vi "RNN_Backward_Pass_demo_alt.vi"() -> ()   [LabVIEW 2014]
uses:
  <vilib>/Analysis/Matrix/Datatypes/RealMatrix.ctl
  <vilib>/Analysis/baseanly.llb/A x Vector.vi
  <vilib>/Analysis/Matrix/Numeric/Conversions/Array To Matrix - RA.vi
  <vilib>/Analysis/Matrix/Numeric/Add/Add - RM,RM.vi
  <vilib>/Analysis/Matrix/NI_Matrix.lvlib
  <vilib>/Analysis/NI_AALBase.lvlib
panel:
  in  "step through t?":bool
  in  "t --->  t - 1":bool
  out "t":i32
  out "t (reversed)":i32
  out "input length":i32=1
  out "dy":dbl[](array[numeric])=[-0.7971630000000001, 0.104457, 0.692257] format="%_8f"
  out "dhnext (out)":dbl[](array[numeric])=[-0.01793824867590542, 0.021743253148573408] format="%_8f"
  out "dhnext (in)":dbl[](array[numeric]) format="%_8f"
  out "dhraw":dbl[](array[numeric])=[0.001989539982402268, -0.041566378972628285] format="%_8f"
  out "dh":dbl[](array[numeric])=[0.24857070126380001, -0.8002550289340001] format="%_8f"
  out "hs[t]":dbl[](array[numeric])=[0.99599, -0.973683] format="%_8f"
  out "hs[t-1]":dbl[](array[numeric]) format="%_8f"
  out "dby":T1=[[-0.7971630000000001], [0.104457], [0.692257]] format="%_8f"
  out "dbh":T1=[[0.001989539982402268], [-0.041566378972628285]] format="%_8f"
  out "dWhy":T1=[[-0.7939663763700001, 0.7761840613290001], [0.10403812743, -0.10170800513099999], [0.68948104943, -0.674038872531]] format="%_8f"
  out "dWhh":T1 format="%_8f"
  out "dWxh":T1=[[0.0, 0.001989539982402268, 0.0], [0.0, -0.041566378972628285, 0.0]] format="%_8f"
  in  "by":T1=[[-0.528417], [-0.44032], [-0.8844819]] format="%_8f"
  in  "bh":T1=[[0.535351], [-1.985987]] format="%_8f"
  in  "Why":T1=[[-0.658616, 0.76469], [-1.7789986, 0.388036], [-0.130912, -0.333988]] format="%_8f"
  in  "Whh":T1=[[-1.3996, 0.961745], [0.364566, -0.477064]] format="%_8f"
  in  "Wxh":T1=[[0.578129, 2.569937, -0.0219857], [-2.46959, 0.027262, 2.4496144]] format="%_8f"
  in  "targets":i32[](array[numeric])=[0]
  in  "hs":dbl[][][](array[numeric])=[[[0.0], [0.0]], [[0.995992], [-0.960992]]] format="%_8f"
  in  "ps":dbl[][][](array[numeric])=[[[0.203285], [0.104457], [0.692257]]] format="%_8f"
  in  "xs":dbl[][][](array[numeric])=[[[0.0], [1.0], [0.0]]]
  in  "inputs":i32[](array[numeric])=[1]
  # "temporary variables"
  # "dParams"
  # "Params"
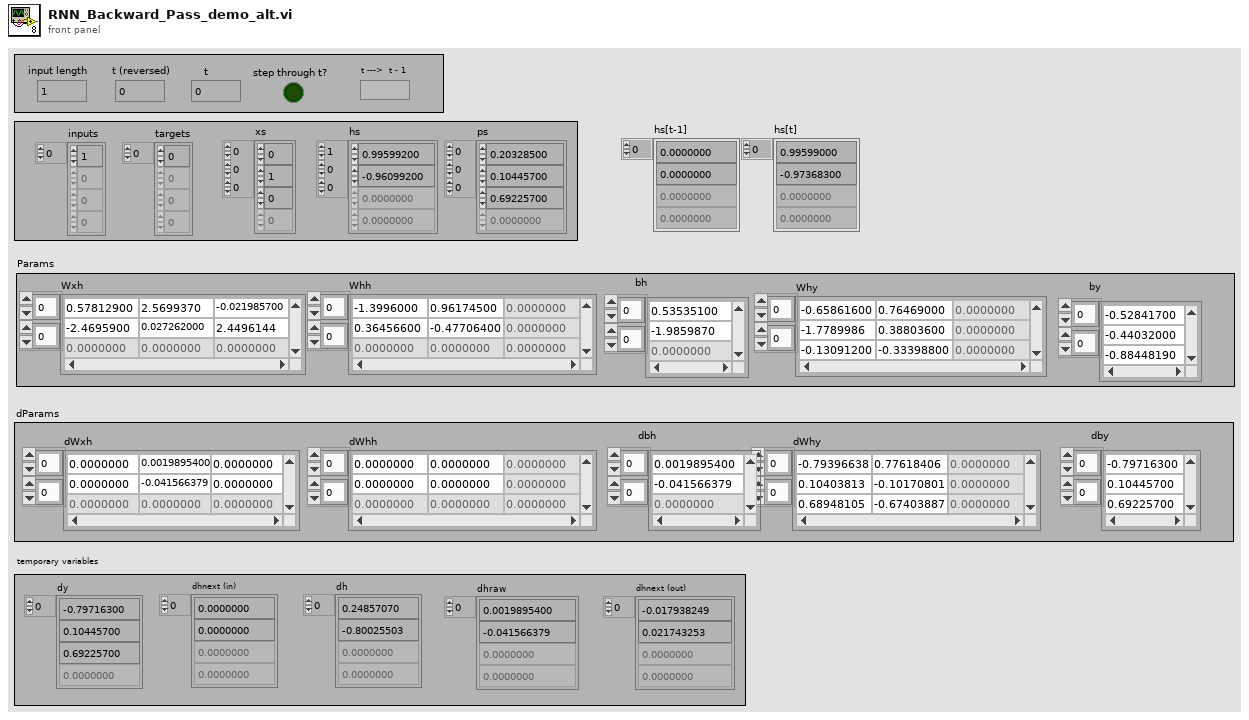
[diagram p1: front panel]
types:
  T1 = typedef "NI_Matrix.lvlib/RealMatrix.ctl" = dbl[][]
  T2 = cluster{"Real Matrix":T1, "Real Matrix":T1, "Real Matrix (Column Vector)":T1, "Real Matrix":T1, "Real Matrix (Column Vector)":T1}
  T3 = cluster{"A + B":T1, "A + B":T1, "Real Matrix (Column Vector)":T1, "A + B":T1, "Real Matrix (Column Vector)":T1}
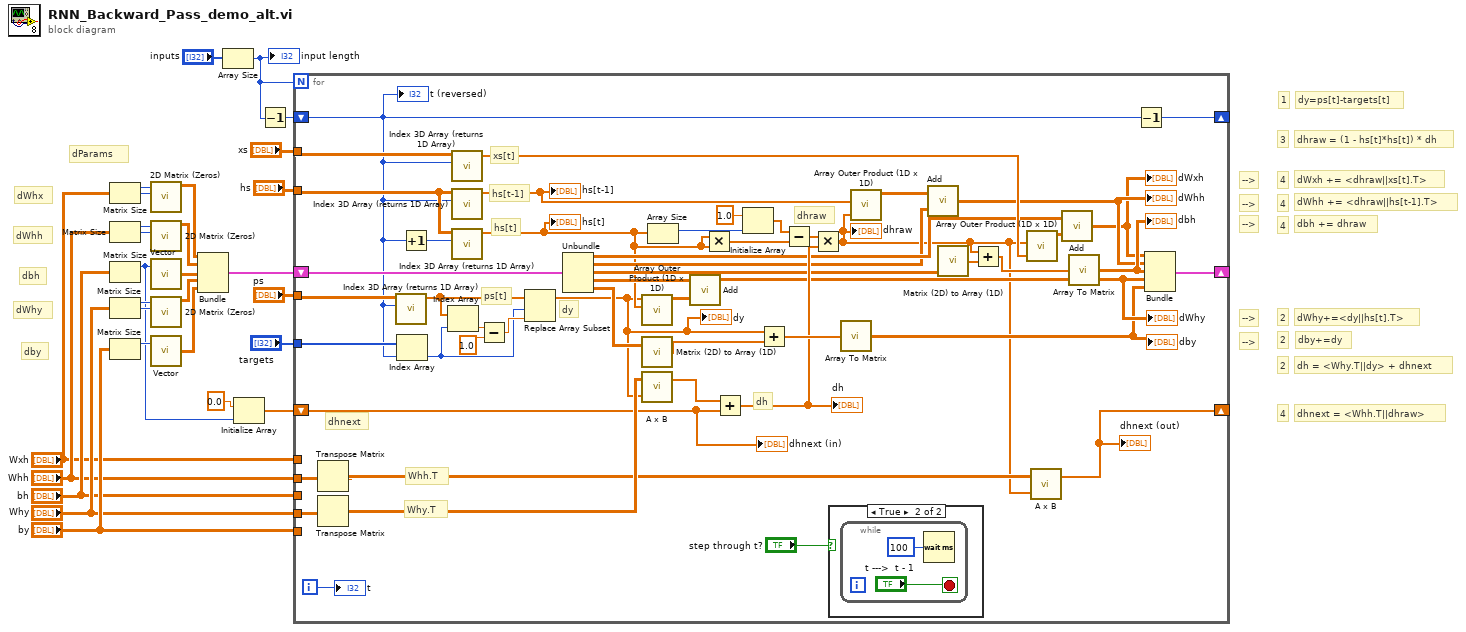
[diagram p0: block diagram]
diagram:
  # "-->"
  # "-->"
  # "-->"
  # "-->"
  # "-->"
  # "4"
  # "4"
  # "4"
  # "4"
  # "3"
  # "2"
  # "2"
  # "2"
  # "1"
  # "dy=ps[t]-targets[t]"
  # "dWhh += <dhraw||hs[t-1].T>"
  # "dby+=dy"
  # "dWhx"
  # "dWhh"
  # "dby"
  # "dWhy"
  # "dbh"
  # "dParams"
  # "dhnext = <Whh.T||dhraw>"
  # "dWxh += <dhraw||xs[t].T>"
  # "dbh += dhraw"
  # "dhraw = (1 - hs[t]*hs[t]) * dh"
  # "dh = <Why.T||dy> + dhnext"
  # "dWhy+=<dy||hs[t].T>"
  n1 = Matrix Size(0:"Wxh") -> (1:w14:i32, 2:w13:i32)
  n2 = Matrix Size(0:"Whh") -> (1:w16:i32, 2:w15:i32)
  n3 = Matrix Size(0:"bh") -> (1:w3:i32)  [unwired: 1 out]
  n4 = Matrix Size(0:"Why") -> (1:w18:i32, 2:w17:i32)
  n5 = Matrix Size(0:"by") -> (1:w19:i32)  [unwired: 1 out]
  n6 = call "2D Matrix (Zeros).vi"("nCols (1)"=w13, "nRows"=w14) -> ("Real Matrix"=w4:T1)  [unwired: 9 in]
  n7 = call "2D Matrix (Zeros).vi"("nCols (1)"=w15, "nRows"=w16) -> ("Real Matrix"=w5:T1)  [unwired: 9 in]
  n8 = call "Vector.vi"("length"=w3) -> ("Real Matrix (Column Vector)"=w6:T1)  [unwired: 1 in]
  n9 = call "2D Matrix (Zeros).vi"("nCols (1)"=w17, "nRows"=w18) -> ("Real Matrix"=w7:T1)  [unwired: 9 in]
  n10 = call "Vector.vi"("length"=w19) -> ("Real Matrix (Column Vector)"=w8:T1)  [unwired: 1 in]
  n11 = Bundle("Real Matrix"=w4, "Real Matrix"=w5, "Real Matrix (Column Vector)"=w6, "Real Matrix"=w7, "Real Matrix (Column Vector)"=w8) -> (w23:T2)  [unwired: 1 in]
  n12 = Array Size(array="inputs") -> (size(s)=w22:i32)
  "input length" <- w22
  n13 = Initialize Array(0.0 ("element"), w3) -> (w1:dbl[])
  n14 = Decrement(x=w22) -> (x-1=w21:i32)
  n15 = for {
    N: w22 -> [_]
    shift-right: [w47] -> _
    shift-left: w23 -> [w66]
    tunnel: "xs" -> [w76]
    tunnel: "hs" -> [w74]
    tunnel: "ps" -> [w75]
    shift-right: [w78] -> _
    shift-left: w21 -> [w43]
    tunnel: "targets" -> [w77]
    shift-right: [w30] -> _
    shift-left: w1 -> [w34]
    tunnel: "Why" -> [w46]
    tunnel: "Whh" -> [w45]
    tunnel: "Wxh" -> [_]
    tunnel: "by" -> [_]
    tunnel: "bh" -> [_]
    i -> [w79]
    # "dhnext"
    # "Whh.T"
    # "dy"
    # "dhraw"
    # "dh"
    # "Why.T"
    # "hs[t-1]"
    # "hs[t]"
    # "xs[t]"
    # "ps[t]"
    n16 = Transpose Matrix(1:w45) -> (0:w50:T1)
    n17 = Transpose Matrix(1:w46) -> (0:w62:T1)
    n18 = call "Index 3D Array (returns 1D Array).vi"("index"=w43, "3D array"=w75) -> ("1D array"=w71:dbl[])  [unwired: 9 in]
    n19 = Index Array(array=w77, index=w43) -> (element=w69:i32)
    n20 = Increment(x=w43) -> (x+1=w44:i32)
    n21 = Index Array(array=w71, index=w69) -> (element=w73:dbl)
    n22 = call "Index 3D Array (returns 1D Array).vi"("index"=w43, "3D array"=w76) -> ("1D array"=w53:dbl[])  [unwired: 9 in]
    n23 = call "Index 3D Array (returns 1D Array).vi"("index"=w43, "3D array"=w74) -> ("1D array"=w49:dbl[])  [unwired: 9 in]
    "hs[t-1]" <- w49
    n24 = call "Index 3D Array (returns 1D Array).vi"("index"=w44, "3D array"=w74) -> ("1D array"=w32:dbl[])  [unwired: 9 in]
    "hs[t]" <- w32
    n25 = Subtract(x=w73, y=1.0) -> (x-y=w70:dbl)
    n26 = Replace Array Subset(array=w71, new element=w70, index=w69) -> (w31:dbl[])
    "dy" <- w31
    n27 = Unbundle(w66) -> ("Real Matrix"=w52:T1, "Real Matrix"=w37:T1, "Real Matrix (Column Vector)"=w54:T1, "Real Matrix"=w64:T1, "Real Matrix (Column Vector)"=w65:T1)
    n28 = call "Array Outer Product (1D x 1D).vi"("array b"=w32, "array a"=w31) -> ("a X b"=w63:dbl[][])  [unwired: 9 in]
    n29 = call "Matrix (2D) to Array (1D).vi"("Matrix (2D)"=w65) -> ("Array (1D)"=w67:dbl[])  [unwired: 4 in]
    n30 = call-poly <vilib>:"A x B.vi"("Vector"=w31, "A"=w62) -> ("A x Vector"=w61:dbl[])  [unwired: 1 out]
    n31 = Array Size(array=w32) -> (size(s)=w60:i32)
    n32 = call-poly <vilib>:"Add.vi"("Real Matrix B"=w63, "Real Matrix A"=w64) -> ("A + B"=w42:T1)
    "dWhy" <- w42
    n33 = Multiply(x=w32, y=w32) -> (x*y=w57:dbl[])
    n34 = Add ("Add.vi")(x=w61, y=w34) -> (x+y=w56:dbl[])
    "dh" <- w56
    n35 = Initialize Array(1.0 ("element"), w60) -> (w58:dbl[])
    n36 = Add(x=w31, y=w67) -> (x+y=w68:dbl[])
    n37 = Subtract(x=w58, y=w57) -> (x-y=w55:dbl[])
    n38 = Multiply(x=w55, y=w56) -> (x*y=w33:dbl[])
    "dhraw" <- w33
    n39 = case shown="True" "step through t?" {
      frame False {
      }
      frame True {
        n40 = while {
          stop <- "t --->  t - 1" stop-if-true
          n41 = Wait (ms)(milliseconds to wait=u32 100) -> ()  [unwired: 1 out]
        }
      }
    }
    n42 = call-poly <vilib>:"Array To Matrix.vi"("Real 1D Array"=w68) -> ("Real Matrix (Column Vector)"=w41:T1)
    "dby" <- w41
    n43 = call "Array Outer Product (1D x 1D).vi"("array b"=w49, "array a"=w33) -> ("a X b"=w36:dbl[][])  [unwired: 9 in]
    n44 = call-poly <vilib>:"Add.vi"("Real Matrix B"=w37, "Real Matrix A"=w36) -> ("A + B"=w39:T1)
    "dWhh" <- w39
    n45 = call "Matrix (2D) to Array (1D).vi"("Matrix (2D)"=w54) -> ("Array (1D)"=w35:dbl[])  [unwired: 4 in]
    n46 = Add ("Add.vi")(x=w33, y=w35) -> (x+y=w48:dbl[])
    n47 = call "Array Outer Product (1D x 1D).vi"("array b"=w53, "array a"=w33) -> ("a X b"=w51:dbl[][])  [unwired: 9 in]
    n48 = call-poly <vilib>:"A x B.vi"("Vector"=w33, "A"=w50) -> ("A x Vector"=w30:dbl[])  [unwired: 1 out]
    "dhnext (out)" <- w30
    n49 = call-poly <vilib>:"Add.vi"("Real Matrix B"=w51, "Real Matrix A"=w52) -> ("A + B"=w38:T1)
    "dWxh" <- w38
    n50 = call-poly <vilib>:"Array To Matrix.vi"("Real 1D Array"=w48) -> ("Real Matrix (Column Vector)"=w40:T1)
    "dbh" <- w40
    n51 = Decrement(x=w43) -> (x-1=w78:i32)
    n52 = Bundle("A + B"=w38, "A + B"=w39, "Real Matrix (Column Vector)"=w40, "A + B"=w42, "Real Matrix (Column Vector)"=w41) -> (w47:T3)  [unwired: 1 in]
    "t" <- w79
    "t (reversed)" <- w43
    "dhnext (in)" <- w34
  }
